vi "lxw datetime to excel datetime.vi"(8 "error in (no error)":errorcluster, 11 "datetime":T1) -> (0 "error out":errorcluster, 2 "function return":dbl, 3 "datetime out":T1)   [LabVIEW 2015, in "xlsxwriter.lvlib"]
doc: "double lxw_datetime_to_excel_datetime(lxw_datetime *datetime);"
uses:
  xlsxwriter.lvlib
  xlsxwriter.dll
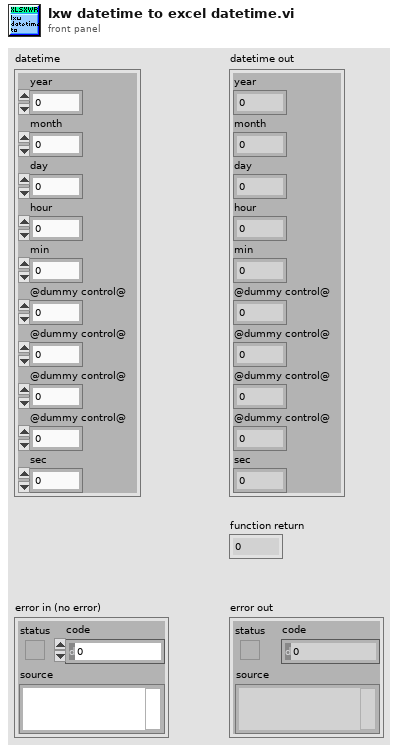
[diagram p1: front panel]
types:
  T1 = cluster{"year":i32, "month":i32, "day":i32, "hour":i32, "min":i32, "@dummy control@":i8, "@dummy control@":i8, "@dummy control@":i8, "@dummy control@":i8, "sec":dbl}
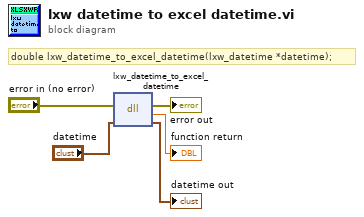
[diagram p0: block diagram]
diagram:
  # "double lxw_datetime_to_excel_datetime(lxw_datetime *datetime);"
  n1 = dll-call lib="C:/Users/WDAGUtilityAccount/Desktop/lv_vis_added_cell/xlsxwriter.*" fn="lxw_datetime_to_excel_datetime"(error in="error in (no error)", "datetime"="datetime") -> (error out=→"error out":errorcluster, →"function return":dbl, "datetime"=→"datetime out":T1)  [unwired: 2 in, 1 out]
